vi "Konvertieren.vi"(10 "Regler":T2[](array[typedef]) {"Error" format="%#.0f"; "Status" format="%#.0f"; "Stellgröße" format="%#.0f"; "Sollwert" format="%#.0f"; "Istwert" format="%#.0f"}, 11 "Grenzwerte PNS (Eingang)":T3 {"Heizleitung 12:"."Regler" items=["aktiv", "inaktiv"]; "Heizleitung 12:"."Abschalt-Max" format="%#_5g"; "Heizleitung 12:"."Abschalt-Min" format="%#_5g"; "Heizleitung 12:"."Warn-Max" format="%#_5g"; "Heizleitung 12:"."Warn-Min" format="%#_5g"; "Heizleitung 12:"."Sollwert" format="%#_5g"; "Heizleitung 11:"."Regler" items=["aktiv", "inaktiv"]; "Heizleitung 11:"."Abschalt-Max" format="%#_5g"; "Heizleitung 11:"."Abschalt-Min" format="%#_5g"; "Heizleitung 11:"."Warn-Max" format="%#_5g"; "Heizleitung 11:"."Warn-Min" format="%#_5g"; "Heizleitung 11:"."Sollwert" format="%#_5g"; "Heizleitung 10:"."Regler" items=["aktiv", "inaktiv"]; "Heizleitung 10:"."Abschalt-Max" format="%#_5g"; "Heizleitung 10:"."Abschalt-Min" format="%#_5g"; "Heizleitung 10:"."Warn-Max" format="%#_5g"; "Heizleitung 10:"."Warn-Min" format="%#_5g"; "Heizleitung 10:"."Sollwert" format="%#_5g"; "Heizleitung 9:"."Regler" items=["aktiv", "inaktiv"]; "Heizleitung 9:"."Abschalt-Max" format="%#_5g"; "Heizleitung 9:"."Abschalt-Min" format="%#_5g"; "Heizleitung 9:"."Warn-Max" format="%#_5g"; "Heizleitung 9:"."Warn-Min" format="%#_5g"; "Heizleitung 9:"."Sollwert" format="%#_5g"; "Heizleitung 8:"."Regler" items=["aktiv", "inaktiv"]; "Heizleitung 8:"."Abschalt-Max" format="%#_5g"; "Heizleitung 8:"."Abschalt-Min" format="%#_5g"; "Heizleitung 8:"."Warn-Max" format="%#_5g"; "Heizleitung 8:"."Warn-Min" format="%#_5g"; "Heizleitung 8:"."Sollwert" format="%#_5g"; "Heizleitung 7:"."Regler" items=["aktiv", "inaktiv"]; "Heizleitung 7:"."Abschalt-Max" format="%#_5g"; "Heizleitung 7:"."Abschalt-Min" format="%#_5g"; "Heizleitung 7:"."Warn-Max" format="%#_5g"; "Heizleitung 7:"."Warn-Min" format="%#_5g"; "Heizleitung 7:"."Sollwert" format="%#_5g"; "Heizleitung 6:"."Regler" items=["aktiv", "inaktiv"]; "Heizleitung 6:"."Abschalt-Max" format="%#_5g"; "Heizleitung 6:"."Abschalt-Min" format="%#_5g"; "Heizleitung 6:"."Warn-Max" format="%#_5g"; "Heizleitung 6:"."Warn-Min" format="%#_5g"; "Heizleitung 6:"."Sollwert" format="%#_5g"; "Heizleitung 5:"."Regler" items=["aktiv", "inaktiv"]; "Heizleitung 5:"."Abschalt-Max" format="%#_5g"; "Heizleitung 5:"."Abschalt-Min" format="%#_5g"; "Heizleitung 5:"."Warn-Max" format="%#_5g"; "Heizleitung 5:"."Warn-Min" format="%#_5g"; "Heizleitung 5:"."Sollwert" format="%#_5g"; "Heizleitung 4:"."Regler" items=["aktiv", "inaktiv"]; "Heizleitung 4:"."Abschalt-Max" format="%#_5g"; "Heizleitung 4:"."Abschalt-Min" format="%#_5g"; "Heizleitung 4:"."Warn-Max" format="%#_5g"; "Heizleitung 4:"."Warn-Min" format="%#_5g"; "Heizleitung 4:"."Sollwert" format="%#_5g"; "Heizleitung 3:"."Regler" items=["aktiv", "inaktiv"]; "Heizleitung 3:"."Abschalt-Max" format="%#_5g"; "Heizleitung 3:"."Abschalt-Min" format="%#_5g"; "Heizleitung 3:"."Warn-Max" format="%#_5g"; "Heizleitung 3:"."Warn-Min" format="%#_5g"; "Heizleitung 3:"."Sollwert" format="%#_5g"; "Heizleitung 2:"."Regler" items=["aktiv", "inaktiv"]; "Heizleitung 2:"."Abschalt-Max" format="%#_5g"; "Heizleitung 2:"."Abschalt-Min" format="%#_5g"; "Heizleitung 2:"."Warn-Max" format="%#_5g"; "Heizleitung 2:"."Warn-Min" format="%#_5g"; "Heizleitung 2:"."Sollwert" format="%#_5g"; "Heizleitung 1:"."Regler" items=["aktiv", "inaktiv"]; "Heizleitung 1:"."Abschalt-Max" format="%#_5g"; "Heizleitung 1:"."Abschalt-Min" format="%#_5g"; "Heizleitung 1:"."Warn-Max" format="%#_5g"; "Heizleitung 1:"."Warn-Min" format="%#_5g"; "Heizleitung 1:"."Sollwert" format="%#_5g"; "Ventilplatte:"."Regler" items=["aktiv", "inaktiv"]; "Ventilplatte:"."Abschalt-Max" format="%#_5g"; "Ventilplatte:"."Abschalt-Min" format="%#_5g"; "Ventilplatte:"."Warn-Max" format="%#_5g"; "Ventilplatte:"."Warn-Min" format="%#_5g"; "Ventilplatte:"."Sollwert" format="%#_5g"; "Filter:"."Regler" items=["aktiv", "inaktiv"]; "Filter:"."Abschalt-Max" format="%#_5g"; "Filter:"."Abschalt-Min" format="%#_5g"; "Filter:"."Warn-Max" format="%#_5g"; "Filter:"."Warn-Min" format="%#_5g"; "Filter:"."Sollwert" format="%#_5g"}) -> (2 "Grenzwerte PNS (Ausgang)":T3 {"Heizleitung 12:"."Regler" items=["aktiv", "inaktiv"]; "Heizleitung 12:"."Abschalt-Max" format="%#_5g"; "Heizleitung 12:"."Abschalt-Min" format="%#_5g"; "Heizleitung 12:"."Warn-Max" format="%#_5g"; "Heizleitung 12:"."Warn-Min" format="%#_5g"; "Heizleitung 12:"."Sollwert" format="%#_5g"; "Heizleitung 11:"."Regler" items=["aktiv", "inaktiv"]; "Heizleitung 11:"."Abschalt-Max" format="%#_5g"; "Heizleitung 11:"."Abschalt-Min" format="%#_5g"; "Heizleitung 11:"."Warn-Max" format="%#_5g"; "Heizleitung 11:"."Warn-Min" format="%#_5g"; "Heizleitung 11:"."Sollwert" format="%#_5g"; "Heizleitung 10:"."Regler" items=["aktiv", "inaktiv"]; "Heizleitung 10:"."Abschalt-Max" format="%#_5g"; "Heizleitung 10:"."Abschalt-Min" format="%#_5g"; "Heizleitung 10:"."Warn-Max" format="%#_5g"; "Heizleitung 10:"."Warn-Min" format="%#_5g"; "Heizleitung 10:"."Sollwert" format="%#_5g"; "Heizleitung 9:"."Regler" items=["aktiv", "inaktiv"]; "Heizleitung 9:"."Abschalt-Max" format="%#_5g"; "Heizleitung 9:"."Abschalt-Min" format="%#_5g"; "Heizleitung 9:"."Warn-Max" format="%#_5g"; "Heizleitung 9:"."Warn-Min" format="%#_5g"; "Heizleitung 9:"."Sollwert" format="%#_5g"; "Heizleitung 8:"."Regler" items=["aktiv", "inaktiv"]; "Heizleitung 8:"."Abschalt-Max" format="%#_5g"; "Heizleitung 8:"."Abschalt-Min" format="%#_5g"; "Heizleitung 8:"."Warn-Max" format="%#_5g"; "Heizleitung 8:"."Warn-Min" format="%#_5g"; "Heizleitung 8:"."Sollwert" format="%#_5g"; "Heizleitung 7:"."Regler" items=["aktiv", "inaktiv"]; "Heizleitung 7:"."Abschalt-Max" format="%#_5g"; "Heizleitung 7:"."Abschalt-Min" format="%#_5g"; "Heizleitung 7:"."Warn-Max" format="%#_5g"; "Heizleitung 7:"."Warn-Min" format="%#_5g"; "Heizleitung 7:"."Sollwert" format="%#_5g"; "Heizleitung 6:"."Regler" items=["aktiv", "inaktiv"]; "Heizleitung 6:"."Abschalt-Max" format="%#_5g"; "Heizleitung 6:"."Abschalt-Min" format="%#_5g"; "Heizleitung 6:"."Warn-Max" format="%#_5g"; "Heizleitung 6:"."Warn-Min" format="%#_5g"; "Heizleitung 6:"."Sollwert" format="%#_5g"; "Heizleitung 5:"."Regler" items=["aktiv", "inaktiv"]; "Heizleitung 5:"."Abschalt-Max" format="%#_5g"; "Heizleitung 5:"."Abschalt-Min" format="%#_5g"; "Heizleitung 5:"."Warn-Max" format="%#_5g"; "Heizleitung 5:"."Warn-Min" format="%#_5g"; "Heizleitung 5:"."Sollwert" format="%#_5g"; "Heizleitung 4:"."Regler" items=["aktiv", "inaktiv"]; "Heizleitung 4:"."Abschalt-Max" format="%#_5g"; "Heizleitung 4:"."Abschalt-Min" format="%#_5g"; "Heizleitung 4:"."Warn-Max" format="%#_5g"; "Heizleitung 4:"."Warn-Min" format="%#_5g"; "Heizleitung 4:"."Sollwert" format="%#_5g"; "Heizleitung 3:"."Regler" items=["aktiv", "inaktiv"]; "Heizleitung 3:"."Abschalt-Max" format="%#_5g"; "Heizleitung 3:"."Abschalt-Min" format="%#_5g"; "Heizleitung 3:"."Warn-Max" format="%#_5g"; "Heizleitung 3:"."Warn-Min" format="%#_5g"; "Heizleitung 3:"."Sollwert" format="%#_5g"; "Heizleitung 2:"."Regler" items=["aktiv", "inaktiv"]; "Heizleitung 2:"."Abschalt-Max" format="%#_5g"; "Heizleitung 2:"."Abschalt-Min" format="%#_5g"; "Heizleitung 2:"."Warn-Max" format="%#_5g"; "Heizleitung 2:"."Warn-Min" format="%#_5g"; "Heizleitung 2:"."Sollwert" format="%#_5g"; "Heizleitung 1:"."Regler" items=["aktiv", "inaktiv"]; "Heizleitung 1:"."Abschalt-Max" format="%#_5g"; "Heizleitung 1:"."Abschalt-Min" format="%#_5g"; "Heizleitung 1:"."Warn-Max" format="%#_5g"; "Heizleitung 1:"."Warn-Min" format="%#_5g"; "Heizleitung 1:"."Sollwert" format="%#_5g"; "Ventilplatte:"."Regler" items=["aktiv", "inaktiv"]; "Ventilplatte:"."Abschalt-Max" format="%#_5g"; "Ventilplatte:"."Abschalt-Min" format="%#_5g"; "Ventilplatte:"."Warn-Max" format="%#_5g"; "Ventilplatte:"."Warn-Min" format="%#_5g"; "Ventilplatte:"."Sollwert" format="%#_5g"; "Filter:"."Regler" items=["aktiv", "inaktiv"]; "Filter:"."Abschalt-Max" format="%#_5g"; "Filter:"."Abschalt-Min" format="%#_5g"; "Filter:"."Warn-Max" format="%#_5g"; "Filter:"."Warn-Min" format="%#_5g"; "Filter:"."Sollwert" format="%#_5g"}, 3 "Cluster":T1)   [LabVIEW 2020, in "Amium PNS.lvlib"]
uses:
  Amium PNS.lvlib
  Amium Anlagengrenzwerte PNS.ctl
  Amium Anlagengrenzwerte-Parameter Anzeige.ctl
  Visualisierungs Elemente/Zahlen-Eingabefeld.ctl
  Temperaturregler Cluster.ctl
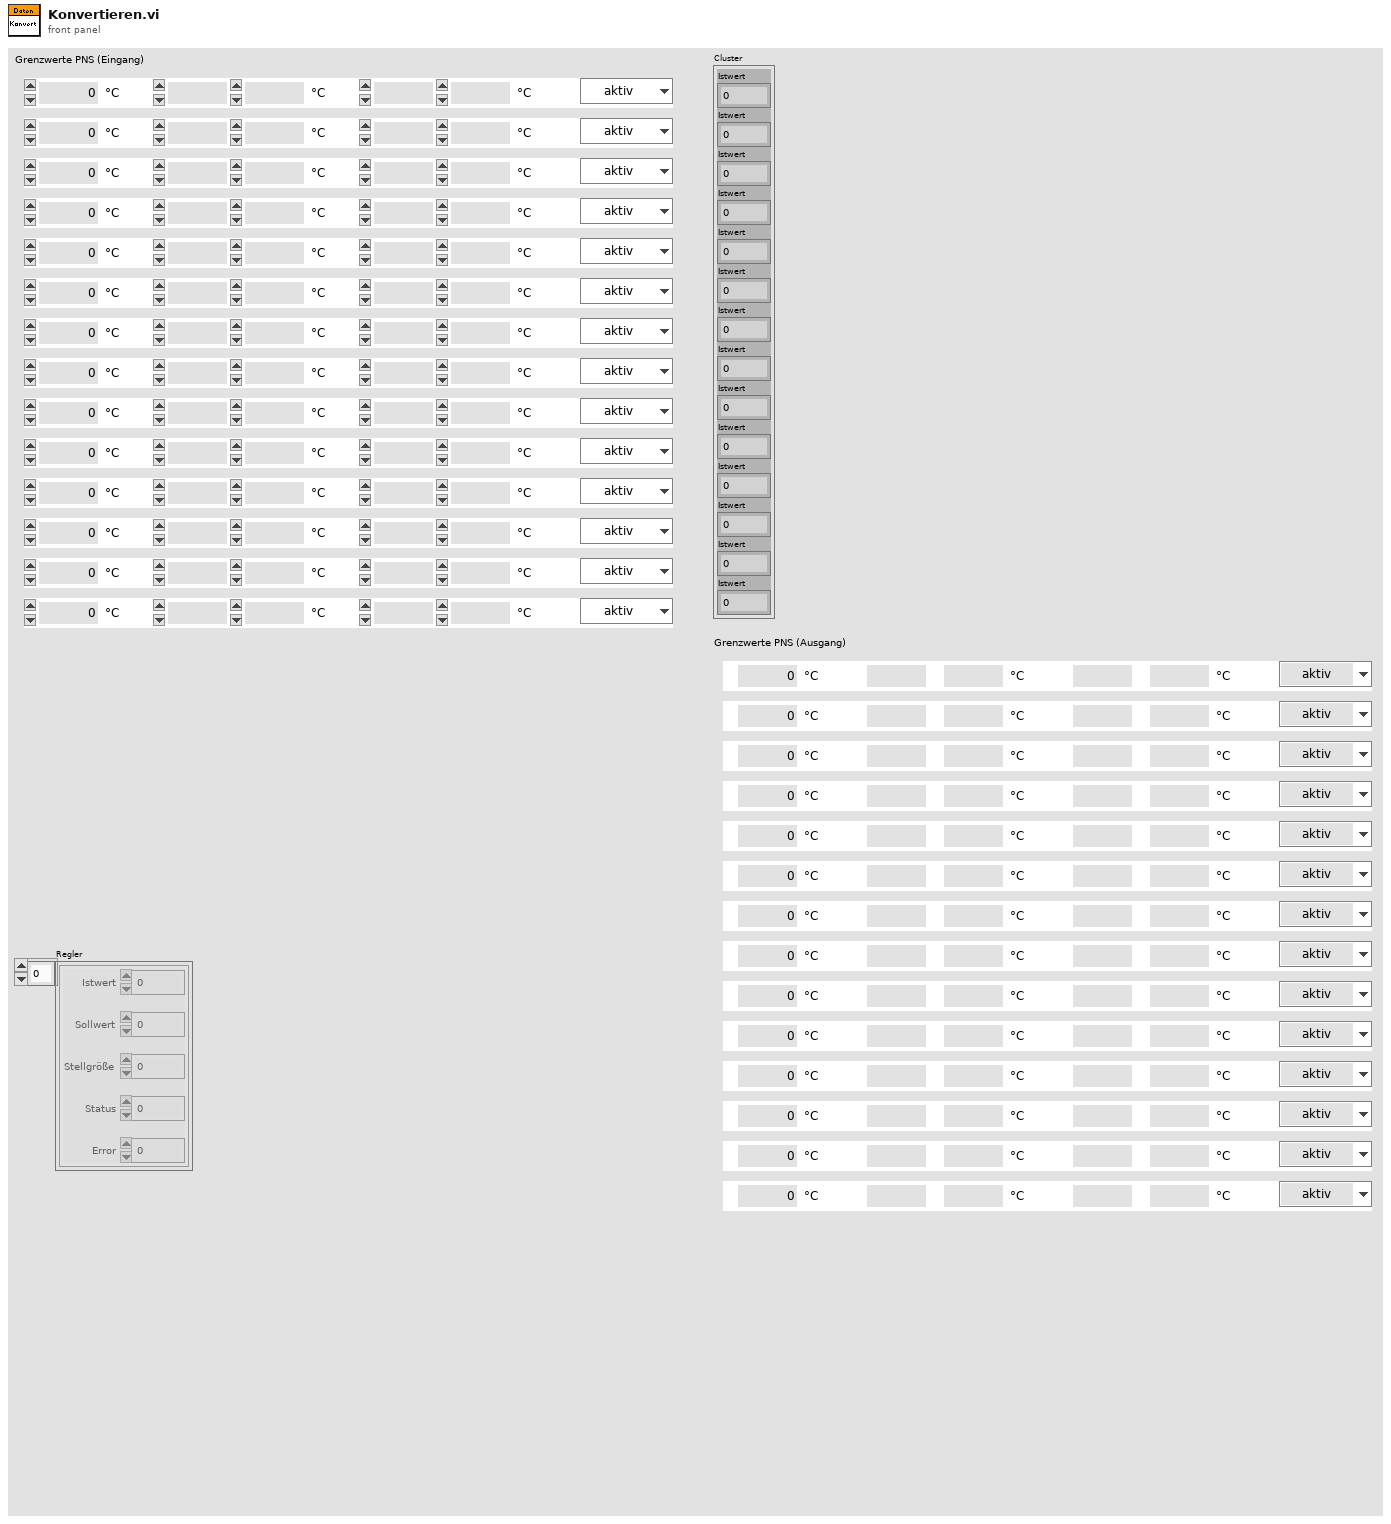
[diagram p1: front panel]
types:
  T1 = cluster{"Istwert":sgl, "Istwert":sgl, "Istwert":sgl, "Istwert":sgl, "Istwert":sgl, "Istwert":sgl, "Istwert":sgl, "Istwert":sgl, "Istwert":sgl, "Istwert":sgl, "Istwert":sgl, "Istwert":sgl, "Istwert":sgl, "Istwert":sgl}
  T2 = typedef "Amium PNS.lvlib/Temperaturregler Cluster.ctl" = cluster{"Istwert":sgl, "Sollwert":sgl, "Stellgröße":sgl, "Status":sgl, "Error":sgl}
  T3 = typedef "Amium PNS.lvlib/Amium Anlagengrenzwerte PNS.ctl" = cluster{"Filter:":T4, "Ventilplatte:":T4, "Heizleitung 1:":T4, "Heizleitung 2:":T4, "Heizleitung 3:":T4, "Heizleitung 4:":T4, "Heizleitung 5:":T4, "Heizleitung 6:":T4, "Heizleitung 7:":T4, "Heizleitung 8:":T4, "Heizleitung 9:":T4, "Heizleitung 10:":T4, "Heizleitung 11:":T4, "Heizleitung 12:":T4}
  T4 = typedef "Amium PNS.lvlib/Amium Anlagengrenzwerte-Parameter Anzeige.ctl" = cluster{"Sollwert":T5, "Warn-Min":T5, "Warn-Max":T5, "Abschalt-Min":T5, "Abschalt-Max":T5, "Regler":u16}
  T5 = typedef "Zahlen-Eingabefeld.ctl" = sgl
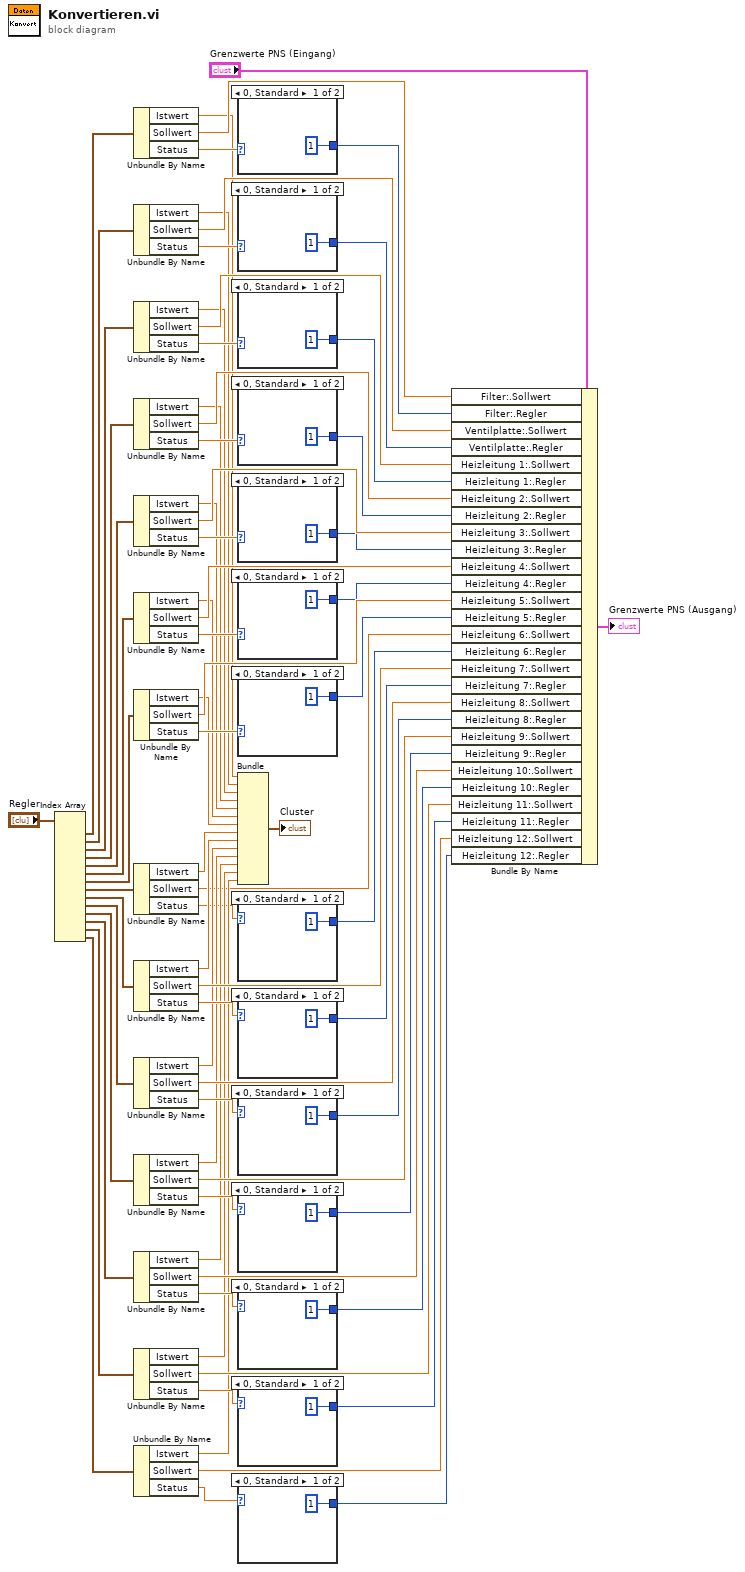
[diagram p0: block diagram]
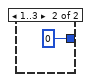
[diagram p2: hidden frame]
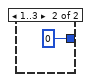
[diagram p3: hidden frame]
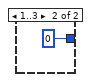
[diagram p4: hidden frame]
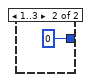
[diagram p5: hidden frame]
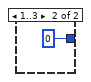
[diagram p6: hidden frame]
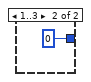
[diagram p7: hidden frame]
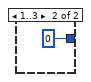
[diagram p8: hidden frame]
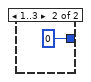
[diagram p9: hidden frame]
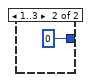
[diagram p10: hidden frame]
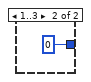
[diagram p11: hidden frame]
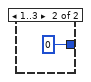
[diagram p12: hidden frame]
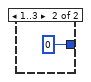
[diagram p13: hidden frame]
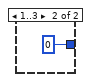
[diagram p14: hidden frame]
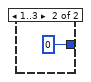
[diagram p15: hidden frame]
diagram:
  n1 = Index Array(array="Regler") -> (element #1=w1:T2, element #2=w2:T2, element #3=w3:T2, element #4=w5:T2, element #5=w4:T2, element #6=w6:T2, element #7=w7:T2, element #8=w15:T2, element #9=w45:T2, element #10=w46:T2, element #11=w47:T2, element #12=w48:T2, element #13=w49:T2, element #14=w50:T2)  [unwired: 14 in]
  n2 = Unbundle By Name(w1) -> ("Istwert"=w8:sgl, "Sollwert"=w37:sgl, "Status"=w25:sgl)
  n3 = Unbundle By Name(w2) -> ("Istwert"=w9:sgl, "Sollwert"=w38:sgl, "Status"=w26:sgl)
  n4 = Unbundle By Name(w3) -> ("Istwert"=w10:sgl, "Sollwert"=w39:sgl, "Status"=w27:sgl)
  n5 = Unbundle By Name(w5) -> ("Istwert"=w11:sgl, "Sollwert"=w40:sgl, "Status"=w28:sgl)
  n6 = Unbundle By Name(w4) -> ("Istwert"=w12:sgl, "Sollwert"=w41:sgl, "Status"=w29:sgl)
  n7 = Unbundle By Name(w6) -> ("Istwert"=w13:sgl, "Sollwert"=w42:sgl, "Status"=w30:sgl)
  n8 = Unbundle By Name(w7) -> ("Istwert"=w14:sgl, "Sollwert"=w43:sgl, "Status"=w32:sgl)
  n9 = Unbundle By Name(w15) -> ("Istwert"=w16:sgl, "Sollwert"=w44:sgl, "Status"=w31:sgl)
  n10 = Unbundle By Name(w45) -> ("Istwert"=w51:sgl, "Sollwert"=w57:sgl, "Status"=w58:sgl)
  n11 = Unbundle By Name(w46) -> ("Istwert"=w52:sgl, "Sollwert"=w60:sgl, "Status"=w62:sgl)
  n12 = Unbundle By Name(w47) -> ("Istwert"=w53:sgl, "Sollwert"=w64:sgl, "Status"=w63:sgl)
  n13 = Unbundle By Name(w48) -> ("Istwert"=w54:sgl, "Sollwert"=w66:sgl, "Status"=w67:sgl)
  n14 = Unbundle By Name(w49) -> ("Istwert"=w55:sgl, "Sollwert"=w69:sgl, "Status"=w70:sgl)
  n15 = Unbundle By Name(w50) -> ("Istwert"=w56:sgl, "Sollwert"=w72:sgl, "Status"=w73:sgl)
  n16 = case shown="0, Standard" w25 {
    tunnel: [1 0] -> w34
    frame 0, Default {
    }
    frame 1..3 {
    }
  }
  n17 = case shown="0, Standard" w26 {
    tunnel: [1 0] -> w20
    frame 0, Default {
    }
    frame 1..3 {
    }
  }
  n18 = case shown="0, Standard" w27 {
    tunnel: [1 0] -> w36
    frame 0, Default {
    }
    frame 1..3 {
    }
  }
  n19 = case shown="0, Standard" w28 {
    tunnel: [1 0] -> w21
    frame 0, Default {
    }
    frame 1..3 {
    }
  }
  n20 = case shown="0, Standard" w29 {
    tunnel: [1 0] -> w22
    frame 0, Default {
    }
    frame 1..3 {
    }
  }
  n21 = case shown="0, Standard" w30 {
    tunnel: [1 0] -> w23
    frame 0, Default {
    }
    frame 1..3 {
    }
  }
  n22 = case shown="0, Standard" w32 {
    tunnel: [1 0] -> w33
    frame 0, Default {
    }
    frame 1..3 {
    }
  }
  n23 = Bundle("Istwert"=w8, "Istwert"=w9, "Istwert"=w10, "Istwert"=w11, "Istwert"=w12, "Istwert"=w13, "Istwert"=w14, "Istwert"=w16, "Istwert"=w51, "Istwert"=w52, "Istwert"=w53, "Istwert"=w54, "Istwert"=w55, "Istwert"=w56) -> (→"Cluster":T1)  [unwired: 1 in]
  n24 = case shown="0, Standard" w31 {
    tunnel: [1 0] -> w24
    frame 0, Default {
    }
    frame 1..3 {
    }
  }
  n25 = case shown="0, Standard" w58 {
    tunnel: [1 0] -> w59
    frame 0, Default {
    }
    frame 1..3 {
    }
  }
  n26 = case shown="0, Standard" w62 {
    tunnel: [1 0] -> w61
    frame 0, Default {
    }
    frame 1..3 {
    }
  }
  n27 = case shown="0, Standard" w63 {
    tunnel: [1 0] -> w65
    frame 0, Default {
    }
    frame 1..3 {
    }
  }
  n28 = case shown="0, Standard" w67 {
    tunnel: [1 0] -> w68
    frame 0, Default {
    }
    frame 1..3 {
    }
  }
  n29 = case shown="0, Standard" w70 {
    tunnel: [1 0] -> w71
    frame 0, Default {
    }
    frame 1..3 {
    }
  }
  n30 = case shown="0, Standard" w73 {
    tunnel: [1 0] -> w74
    frame 0, Default {
    }
    frame 1..3 {
    }
  }
  n31 = Bundle By Name(cluster="Grenzwerte PNS (Eingang)", "Filter:.Sollwert"=w37, "Filter:.Regler"=w34, "Ventilplatte:.Sollwert"=w38, "Ventilplatte:.Regler"=w20, "Heizleitung 1:.Sollwert"=w39, "Heizleitung 1:.Regler"=w36, "Heizleitung 2:.Sollwert"=w40, "Heizleitung 2:.Regler"=w21, "Heizleitung 3:.Sollwert"=w41, "Heizleitung 3:.Regler"=w22, "Heizleitung 4:.Sollwert"=w42, "Heizleitung 4:.Regler"=w23, "Heizleitung 5:.Sollwert"=w43, "Heizleitung 5:.Regler"=w33, "Heizleitung 6:.Sollwert"=w44, "Heizleitung 6:.Regler"=w24, "Heizleitung 7:.Sollwert"=w57, "Heizleitung 7:.Regler"=w59, "Heizleitung 8:.Sollwert"=w60, "Heizleitung 8:.Regler"=w61, "Heizleitung 9:.Sollwert"=w64, "Heizleitung 9:.Regler"=w65, "Heizleitung 10:.Sollwert"=w66, "Heizleitung 10:.Regler"=w68, "Heizleitung 11:.Sollwert"=w69, "Heizleitung 11:.Regler"=w71, "Heizleitung 12:.Sollwert"=w72, "Heizleitung 12:.Regler"=w74) -> (→"Grenzwerte PNS (Ausgang)":T3)
